vi "Gamepad Drive.vi"   [LabVIEW 2014]
types:
  T1 = cluster{"Buttons":cluster{"A":bool, "B":bool, "X":bool, "Y":bool, "L Bumper":bool, "R Bumper":bool, "Back":bool, "Start":bool, "LStick":bool, "RStick":bool}, "Axes":cluster{"Left Stick":cluster{"X":dbl, "Y":dbl}, "Right Stick":cluster{"X":dbl, "Y":dbl}, "Triggers":dbl}}
  T2 = cluster{"Left Stick":cluster{"X":dbl, "Y":dbl}, "Right Stick":cluster{"X":dbl, "Y":dbl}, "Triggers":dbl}
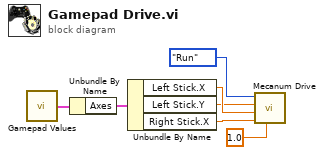
[diagram p0: block diagram]
diagram:
  n1 = call "Gamepad Values.vi"() -> ("Xbox"=w7:T1)
  n2 = Unbundle By Name(w7) -> ("Axes"=w6:T2)
  n3 = Unbundle By Name(w6) -> ("Left Stick.X"=w5:dbl, "Left Stick.Y"=w2:dbl, "Right Stick.X"=w4:dbl)
  n4 = call "Mecanum Drive.vi"("Division"=1.0, "Turn"=w4, "Strafe"=w5, "Forward/Backward"=w2, "Mode"=enum8{"Start", "Run", "Finish"}."Run") -> ()  [unwired: 7 in]
